vi "Construct.vi"(4 "Stale (F)":bool, 6 "Properties":variant, 8 "error in (no error)":errorcluster, 9 "Initial Value":variant, 10 "Name":string, 11 "Tag in":refnum<class "Tag.lvclass">) -> (0 "error out":errorcluster, 3 "Tag out":refnum<class "Tag.lvclass">)   [LabVIEW 2018, in "Tag Engine.lvlib" / "Tag.lvclass"]
doc: "_SubVI_\nInitializes the Tag object.\nThe input initial value will define the type.\n\nThe input Tag name is sanitized. Illegal characters are replaced with underscores.\n\nAdditional properties can be passed in as attributes of the properties varriant."
uses:
  Tag.lvclass
  Types/SetRequest Cluster.ctl
  <vilib>/Utility/Data Type/Type Definitions/Data Type.ctl
  Types/ValChange Cluster.ctl
  Tag.lvclass/Tag.ctl
  Tag Engine.lvlib
  <vilib>/Utility/Data Type/NI_Data Type.lvlib
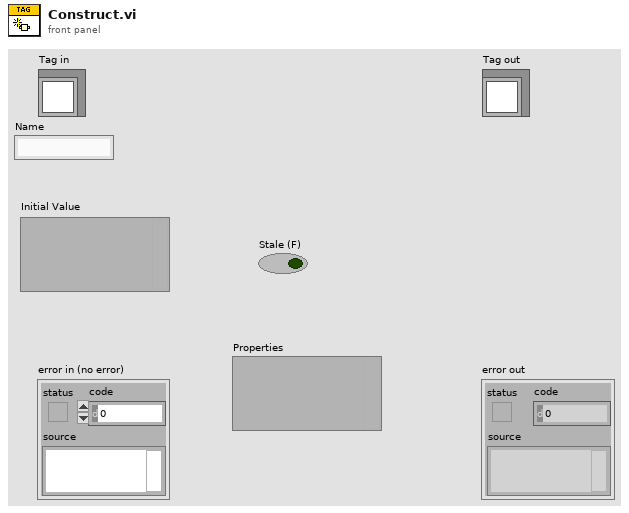
[diagram p1: front panel]
types:
  T1 = typedef "Tag Engine.lvlib/SetRequest Cluster.ctl" = cluster{"Tag Name":string, "Type":T2, "Old Value":variant, "Old Time Stamp":timestamp, "Req Value":variant, "Req Time Stamp":timestamp, "Callback":refnum<notifier>, "Synchronous (F)":bool}
  T2 = typedef "NI_Data Type.lvlib/Data Type.ctl" = enum8{"Invalid Type", "Void", "I8", "I16", "I32", "I64", "U8", "U16", "U32", "U64", "Single Float", "Double Float", "Extended Float", "Single Complex", "Double Complex", "Extended Complex", "Enum U8", "Enum U16", "Enum U32", "Enum U64", "Single Float With Unit", "Double Float With Unit", "Extended Float With Unit", "Single Complex with Unit", "Double Complex with Unit", "Extended Complex with Unit", "Boolean", "String", "Path", "Picture", "Tag", "Array", "Cluster", "Variant", "LV Variant", "Waveform", "Timestamp", "Digital Waveform", "Digital Data", "ExpressData", "Refnum", "External Data", "VI", "Poly VI", "LabVIEW Class Instance", "Fixed Point"}
  T3 = typedef "Tag Engine.lvlib/ValChange Cluster.ctl" = cluster{"Tag Name":string, "Type":T2, "Old Value":variant, "Old Time Stamp":timestamp, "New Value":variant, "New Time Stamp":timestamp}
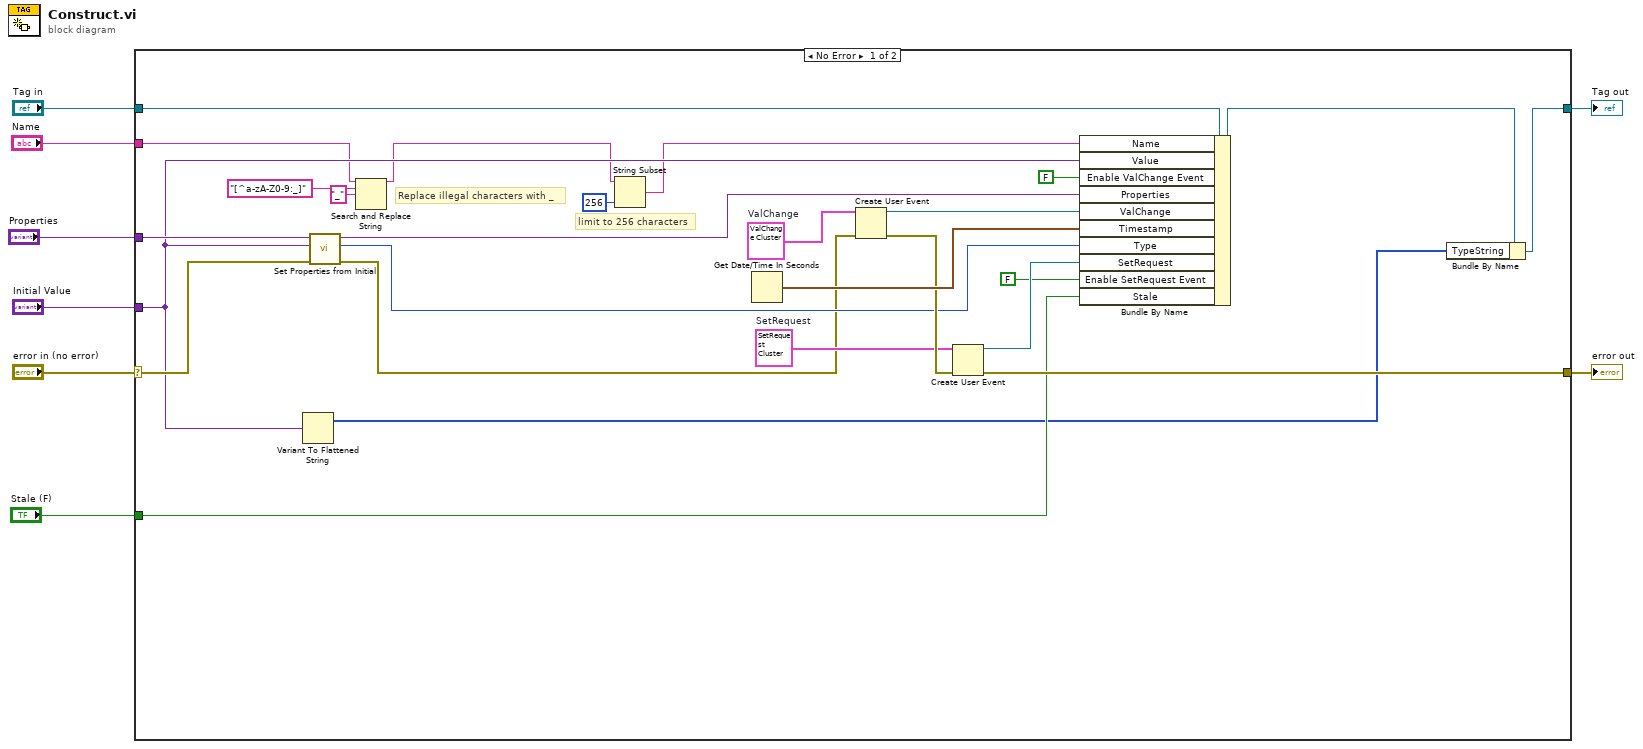
[diagram p0: block diagram]
diagram:
  n1 = case shown="No Error" "error in (no error)" {
    selector: "error in (no error)" -> [w21 w36]
    tunnel: [w29 w36] -> w7
    tunnel: [w17 w35] -> w5
    tunnel: "Tag in" -> [w33 w35]
    tunnel: "Name" -> [w14 _]
    tunnel: "Initial Value" -> [w15 _]
    tunnel: "Properties" -> [w24 _]
    tunnel: "Stale (F)" -> [w19 _]
    frame No Error {
      w27 = T1 {"Tag Name"="", "Type"=enum."Variant", "Old Value"=variant, "Old Time Stamp"=timestamp(0 s since 1904-01-01), "Req Value"=variant, "Req Time Stamp"=timestamp(0 s since 1904-01-01), "Callback"=refnum, "Synchronous (F)"=FALSE}  # SetRequest
      w34 = T3 {"Tag Name"="", "Type"=enum."Variant", "Old Value"=variant, "Old Time Stamp"=timestamp(0 s since 1904-01-01), "New Value"=variant, "New Time Stamp"=timestamp(0 s since 1904-01-01)}  # ValChange
      # "limit to 256 characters"
      # "Replace illegal characters with _"
      n2 = Variant To Flattened String(Variant=w15) -> (1:w16:i16[])  [unwired: 1 out]
      n3 = call "Set Properties from Initial.vi"("error in(no error)"=w21, "Initial Value"=w15, "Properties in"=w24) -> ("error out"=w20:errorcluster, "type"=w22:T2, "Properties out"=w23:variant)  [unwired: 6 in]
      n4 = Search and Replace String(input string=w14, search string="[^a-zA-Z0-9:_]", replace string="_" ("replace string (\"\")")) -> (result string=w10:string)  [unwired: 5 in, 3 out]
      n5 = String Subset(string=w10, length (rest)=256 ("length (rest)")) -> (substring=w9:string)  [unwired: 1 in]
      n6 = Get Date/Time In Seconds() -> (seconds since 1Jan1904=w30:timestamp)
      n7 = Create User Event(user event datatype=w34, error in=w20) -> (user event=w32:refnum<user-event>, error out=w28:errorcluster)
      n8 = Create User Event(user event datatype=w27, error in=w28) -> (user event=w26:refnum<user-event>, error out=w29:errorcluster)
      n9 = Bundle By Name(cluster=w33, "Name"=w9, "Value"=w15, "Enable ValChange Event"=FALSE, "Properties"=w23, "ValChange"=w32, "Timestamp"=w30, "Type"=w22, "SetRequest"=w26, "Enable SetRequest Event"=FALSE, "Stale"=w19) -> (w18:refnum<class "Tag.lvclass">)
      n10 = Bundle By Name(cluster=w18, "TypeString"=w16) -> (w17:refnum<class "Tag.lvclass">)
    }
    frame Error {
    }
  }
  "error out" <- w7
  "Tag out" <- w5
